vi "test tx cmd generation.vi"() -> ()   [LabVIEW 2012]
panel:
  out "RXCommand":string="rx f=5180; r=vt0;  pc=100; ch=0x1; macrx=01.00.00.C0.FF.EE; mactx=01.00.00.C0.FF.EE; bssid=01.00.00.C0.FF.EE; pl=1500; bc=1; ifs=1;"
  in  "AntennaTX4":i32
  in  "AntennaTX2":i32
  in  "AntennaTX3":i32
  in  "AntennaTX1":i32=1
  in  "TxPwrDbm":dbl=17.0
  in  "Bandwidth":string="Legacy"
  in  "DataRate":string="54Mbps"
  in  "Freq":i32=5180
  out "TXCommand":string="tx f=5180;tp=0;pl=1500;pc=100000;r=vt29;ch=1;"
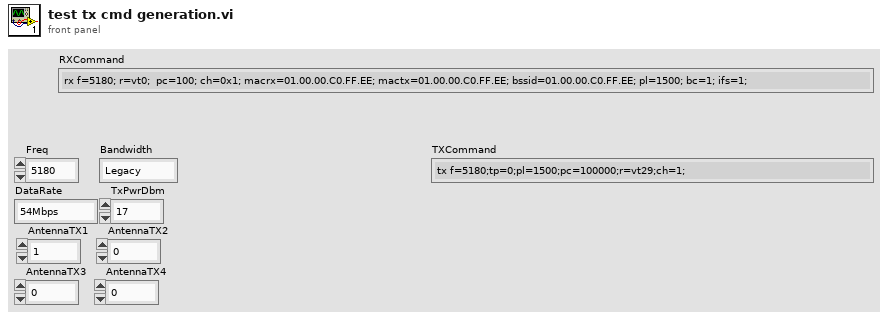
[diagram p1: front panel]
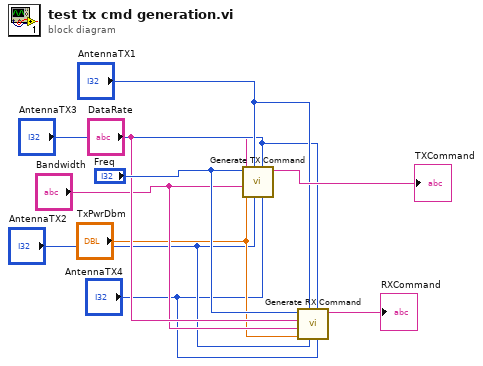
[diagram p0: block diagram]
diagram:
  n1 = call "Generate TX Command.vi"("AntennaTX4"="AntennaTX4", "AntennaTX3"="AntennaTX3", "AntennaTX2"="AntennaTX2", "AntennaTX1"="AntennaTX1", "TxPwrDbm"="TxPwrDbm", "Bandwidth"="Bandwidth", "DataRate"="DataRate", "Freq"="Freq") -> ("TXCommand"=→"TXCommand":string)  [unwired: 3 out]
  n2 = call "Generate RX Command.vi"("AntennaTX4"="AntennaTX4", "AntennaTX3"="AntennaTX3", "AntennaTX2"="AntennaTX2", "AntennaTX1"="AntennaTX1", "RxPwrDbm"="TxPwrDbm", "Bandwidth"="Bandwidth", "DataRate"="DataRate", "Freq"="Freq") -> ("RXCommand"=→"RXCommand":string)  [unwired: 3 out]
